vi "Queue - EnQueue to MessageQ.vi"(8 "Error In (NA)":errorcluster, 9 "<NoD> Don't Display to UI":bool, 11 "Message":string) -> (0 "Error Out":errorcluster)   [LabVIEW 2020]
uses:
  Variables/Global SRTRS.vi
panel:
  in  "<NoML> Don't Update to [MessageLog]":bool
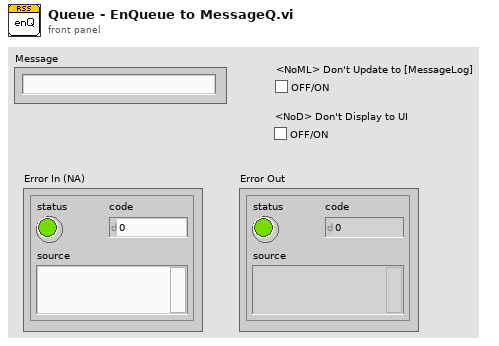
[diagram p1: front panel]
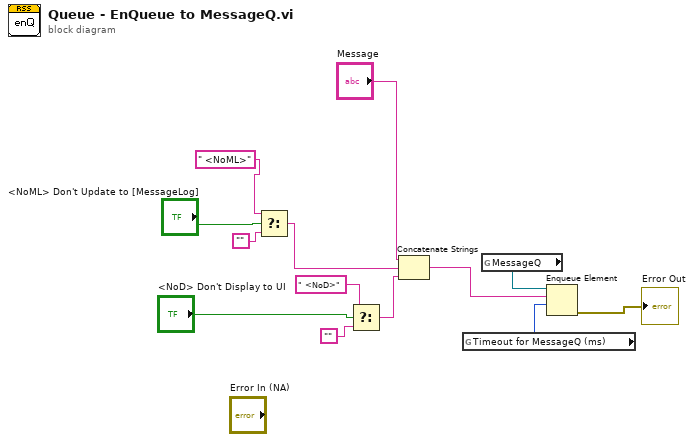
[diagram p0: block diagram]
diagram:
  n1 = Select(t=" <NoML>", s="<NoML> Don't Update to [MessageLog]", f="") -> (s? t:f=w6:string)
  n2 = Select(t=" <NoD>", s="<NoD> Don't Display to UI", f="") -> (s? t:f=w2:string)
  n3 = Concatenate Strings("Message", w6, w2) -> (w5:string)
  n4 = global read "Global SRTRS.vi" "Timeout for MessageQ (ms)"() -> (w13:i32)
  n5 = global read "Global SRTRS.vi" "MessageQ"() -> (w12:refnum<queue>)
  n6 = Enqueue Element(queue=w12, element=w5, timeout in ms (-1)=w13) -> (error out=→"Error Out":errorcluster)  [unwired: 1 in, 2 out]
